vi "gratebar defects finding.vi"(0 "src img path":path, 1 "threshoulds array":dbl[](array[numeric]), 5 "Image":T1, 7 "img out path":path, 9 "size":dbl, 11 "error in (no error)":errorcluster) -> (4 "Image Out (duplicate)":T1, 6 "defect ratio":dbl, 8 "defect type":dbl, 10 "frame statue":dbl, 15 "error out":errorcluster)   [LabVIEW 2014]
uses:
  <vilib>/vision/Image Controls.llb/IMAQ Image.ctl
panel:
  out "size":dbl=5.0
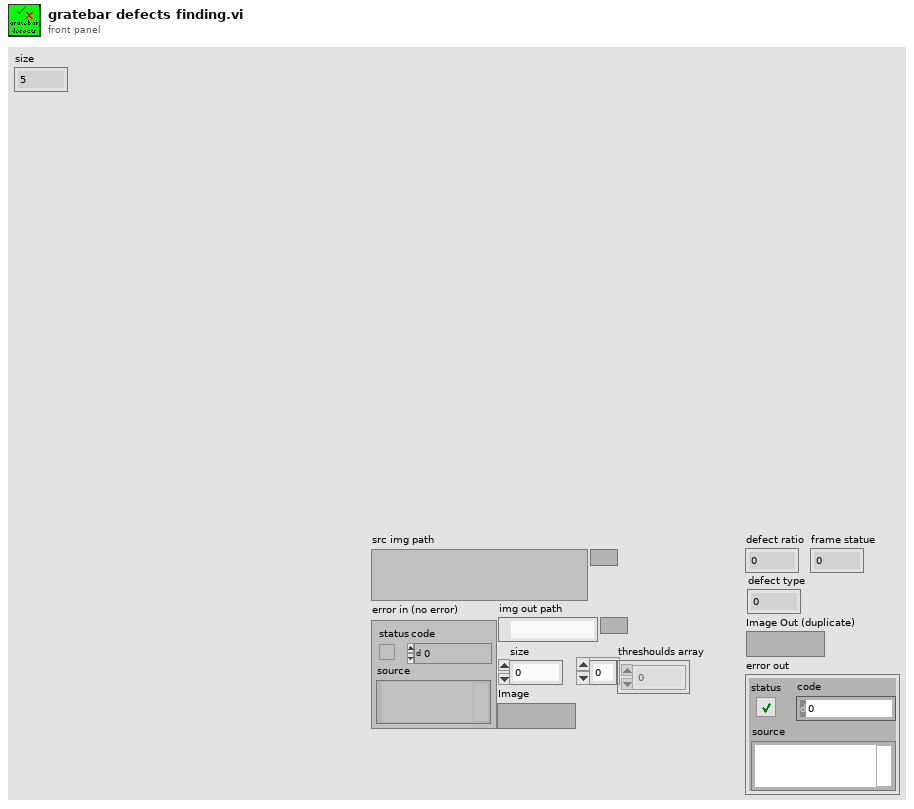
[diagram p1: front panel]
types:
  T1 = typedef "IMAQ Image.ctl" = refnum<image>
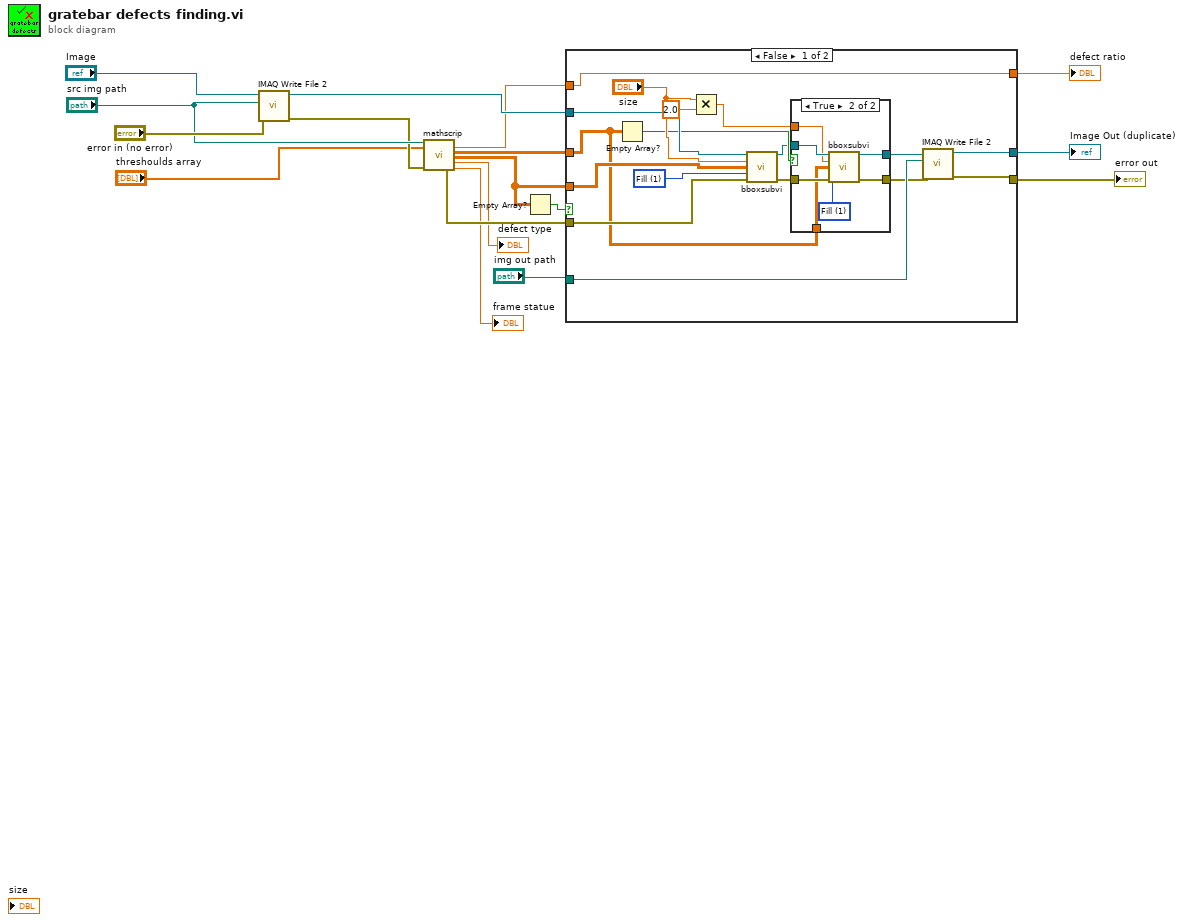
[diagram p0: block diagram]
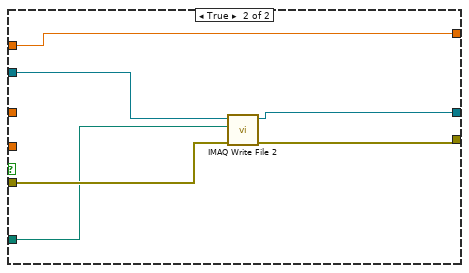
[diagram p3: hidden frame]
diagram:
  n1 = call-poly "IMAQ Write File 2"("error in (no error)"="error in (no error)", "File Path"="src img path", "Image"="Image") -> ("error out"=w8:errorcluster, "Image Out (duplicate)"=w16:T1)  [unwired: 7 in]
  n2 = call "mathscrip.vi"("image path"="src img path", "threshoulds array"="threshoulds array", "error in"=w8) -> ("error out"=w5:errorcluster, "defect ratio1"=w7:dbl, "damage points 2"=w3:dbl[][], "damage points"=w6:dbl[][], "defect type"=→"defect type":dbl, "frame statue"=→"frame statue":dbl)  [unwired: 9 in, 2 out]
  n3 = Empty Array?(array=w6) -> (empty?=w17:bool)
  n4 = case shown="False" w17 {
    tunnel: [w34 w45] -> w11
    tunnel: w6 -> [w29 _]
    tunnel: w5 -> [w28 w48]
    tunnel: "img out path" -> [w33 w47]
    tunnel: [w32 w46] -> w12
    tunnel: w7 -> [w31 w49]
    tunnel: [w31 w49] -> w13
    tunnel: w16 -> [w30 w44]
    tunnel: w3 -> [w20 _]
    frame False {
      w27 = u32 1 items=["Frame", "Fill"] ("Drawing Mode (Frame)")
      n5 = Empty Array?(array=w20) -> (empty?=w24:bool)
      n6 = Multiply(x="size", y=2.0) -> (x*y=w21:dbl)
      n7 = call "bboxsubvi.vi"("Image"=w30, "size"="size", "array"=w29, "Drawing Mode (Frame)"=w27, "error in"=w28) -> ("Image Out"=w23:T1, "error out"=w22:errorcluster)  [unwired: 9 in]
      n8 = case shown="True" w24 {
        tunnel: w23 -> [w36 w43]
        tunnel: w22 -> [w35 w42]
        tunnel: w21 -> [_ w41]
        tunnel: w20 -> [_ w40]
        tunnel: [w36 w38] -> w19
        tunnel: [w35 w37] -> w18
        frame False {
        }
        frame True {
          w39 = u32 1 items=["Frame", "Fill"] ("Drawing Mode (Frame)")
          n9 = call "bboxsubvi.vi"("Image"=w43, "size"=w41, "array"=w40, "Drawing Mode (Frame)"=w39, "error in"=w42) -> ("Image Out"=w38:T1, "error out"=w37:errorcluster)  [unwired: 9 in]
        }
      }
      n10 = call-poly "IMAQ Write File 2"("error in (no error)"=w18, "File Path"=w33, "Image"=w19) -> ("error out"=w34:errorcluster, "Image Out (duplicate)"=w32:T1)  [unwired: 7 in]
    }
    frame True {
      n11 = call-poly "IMAQ Write File 2"("error in (no error)"=w48, "File Path"=w47, "Image"=w44) -> ("error out"=w45:errorcluster, "Image Out (duplicate)"=w46:T1)  [unwired: 7 in]
    }
  }
  "defect ratio" <- w13
  "Image Out (duplicate)" <- w12
  "error out" <- w11
